vi "Laser Device Control.vi"(7 "Calling VI Ref":refnum<vi>) -> ()   [LabVIEW 2020]
uses:
  Laser Device Control Type Defs/Laser Device Control Control.ctl
  Hardware Configuration/Hardware Configuration Controls/Device Type.ctl
  <vilib>/Utility/miscctls.llb/LVPointTypeDef.ctl
  Device Library/Lasers/Laser Controls/Laser Actions.ctl
  Device Manager/Common Device Queue/Common Device Controls/Common Device Actions.ctl
  <vilib>/regexp/Match Regular Expression.xnode
panel:
  in  "Laser 05":T1={"Wavelength (nm)"=0, "Connect Text"="", "Connection"=TRUE, "Laser Status"="", "Emission"=TRUE, "Power (mW)"=0.0, "Settings"=TRUE}
  in  "Laser 04":T1={"Wavelength (nm)"=0, "Connect Text"="", "Connection"=TRUE, "Laser Status"="", "Emission"=TRUE, "Power (mW)"=0.0, "Settings"=TRUE}
  in  "Laser 03":T1={"Wavelength (nm)"=0, "Connect Text"="", "Connection"=TRUE, "Laser Status"="", "Emission"=TRUE, "Power (mW)"=0.0, "Settings"=TRUE}
  in  "Laser 02":T1={"Wavelength (nm)"=0, "Connect Text"="", "Connection"=TRUE, "Laser Status"="", "Emission"=TRUE, "Power (mW)"=0.0, "Settings"=TRUE}
  in  "Laser 01":T1={"Wavelength (nm)"=0, "Connect Text"="", "Connection"=TRUE, "Laser Status"="", "Emission"=TRUE, "Power (mW)"=0.0, "Settings"=TRUE}
  in  "Quit":bool
  # "Status:"
  # "Status:"
  # "Status:"
  # "Status:"
  # "Status:"
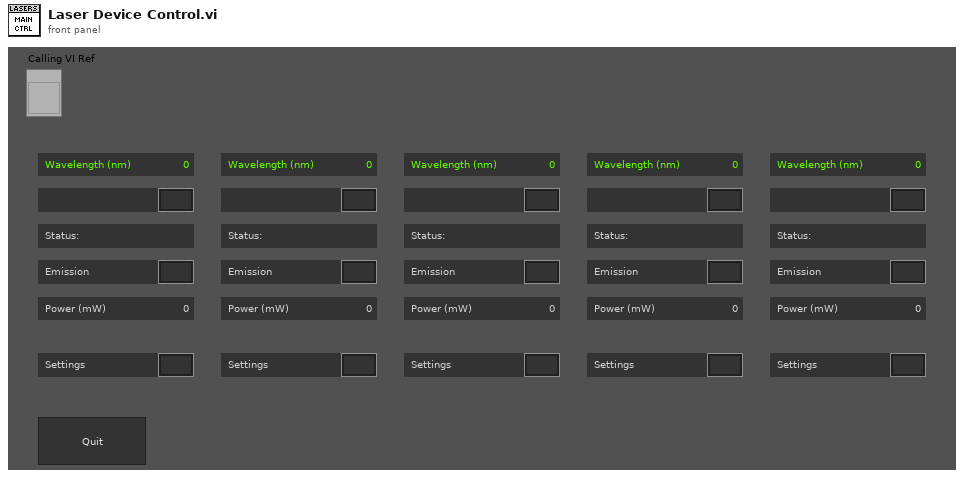
[diagram p1: front panel]
types:
  T1 = typedef "Laser Device Control Control.ctl" = cluster{"Wavelength (nm)":u16, "Connect Text":string, "Connection":bool, "Laser Status":string, "Emission":bool, "Power (mW)":dbl, "Settings":bool}
  T2 = enum16{"Always On", "Always Off", "Off While Running"}
  T3 = typedef "LVPointTypeDef.ctl" = cluster{"Horizontal":i16, "Vertical":i16}
  T4 = typedef "Device Type.ctl" = enum16{"AOTF", "Camera", "Deformable Mirror", "Laser", "Microscope Base", "Shutter", "Stage", "Waveform", "FPGA", "Email", "Filter Wheel", "Spinning Disk"}
  T5 = typedef "LVRectTypeDef.ctl" = cluster{"Left":i16, "Top":i16, "Right":i16, "Bottom":i16}
  T6 = typedef "LVBoundsTypeDef.ctl" = cluster{"Width":u32, "Height":u32}
  T7 = typedef "Laser Actions.ctl" = enum16{"Error Check", "Set On/Off", "Set Power", "Set Parameter", "Get Power", "Get Status", "Get Parameter", "Quit"}
  T8 = typedef "Common Device Actions.ctl" = enum16{"Specific Action", "Open Front Panel", "Close Front Panel", "Quit", "Quit All"}
  T9 = typedef "Laser Control Control.ctl" = cluster{"Wavelength (nm)":u16, "Connect Text":string, "Connection":bool, "Laser Status":string, "Emission":bool, "Power (mW)":dbl, "Settings":bool}
  T10 = typedef "Device Function.ctl" = enum16{"Primary", "Secondary", "Overview", "Wide Field Drift Correction", "642 nm Excitation", "560 nm Excitation", "940 nm Excitation", "546 nm Excitation", "488 nm Excitation", "405 nm Excitation", "Objective Drift Correction", "4Pi Objective Lock", "Objective XY", "Objective Z", "Sample XY", "Sample Coarse Z", "Sample Z", "4Pi Lower", "4Pi Upper", "Mojo", "Adj Cavity", "Line Scanning", "Alert"}
  T11 = typedef "Laser Status.ctl" = enum16{"Warmup", "Ready", "Emission", "Tuning", "Error"}
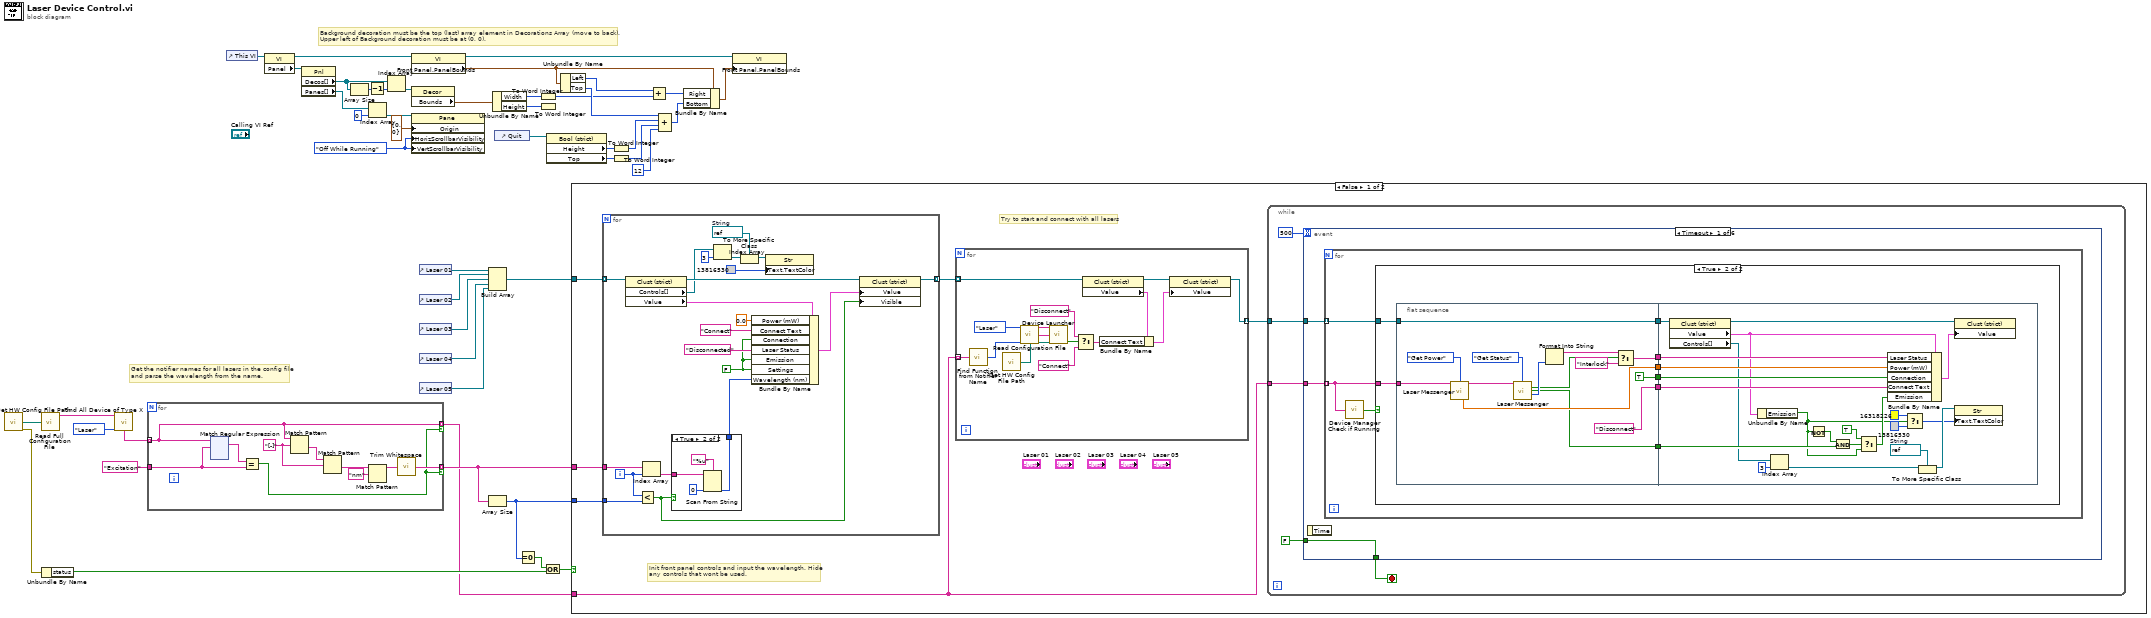
[diagram p0: block diagram]
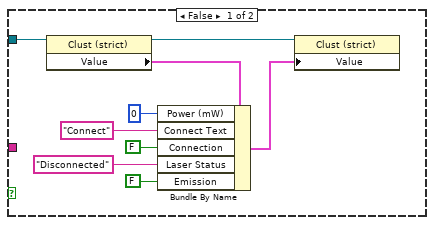
[diagram p2: hidden frame]
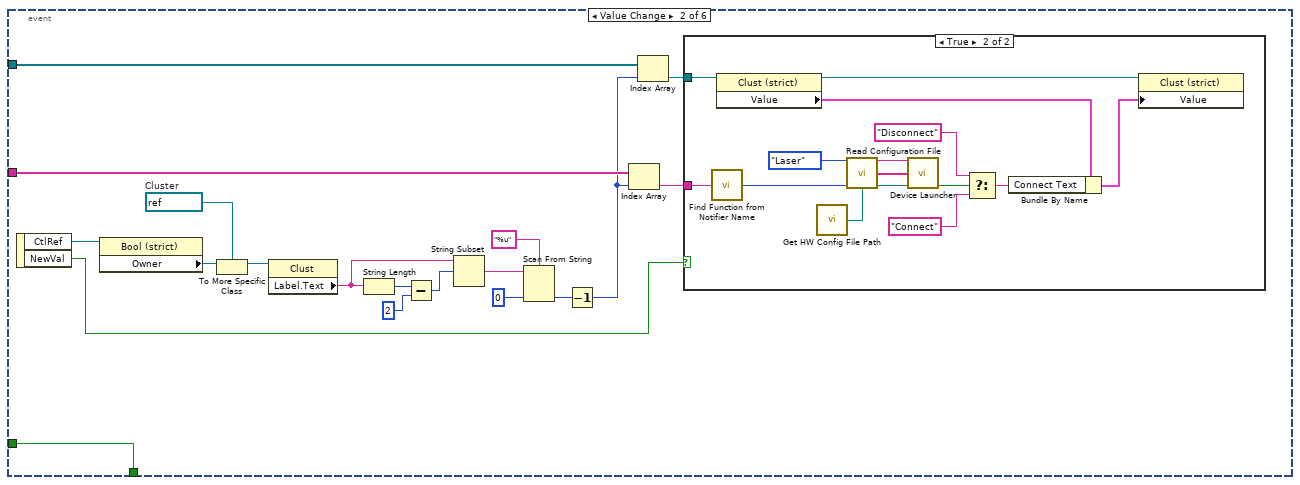
[diagram p3: hidden frame]
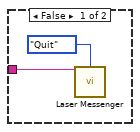
[diagram p4: hidden frame]
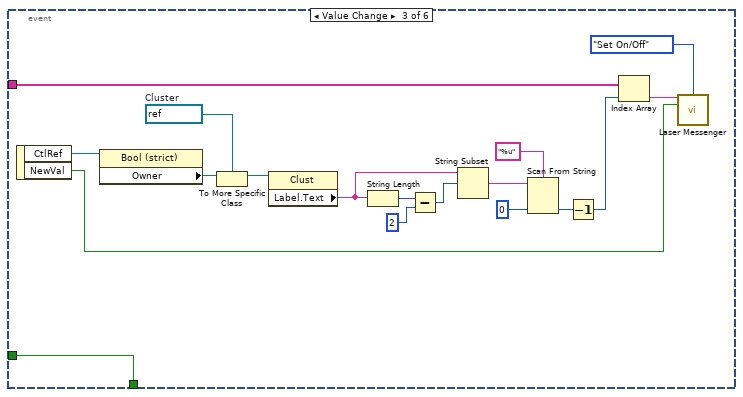
[diagram p5: hidden frame]
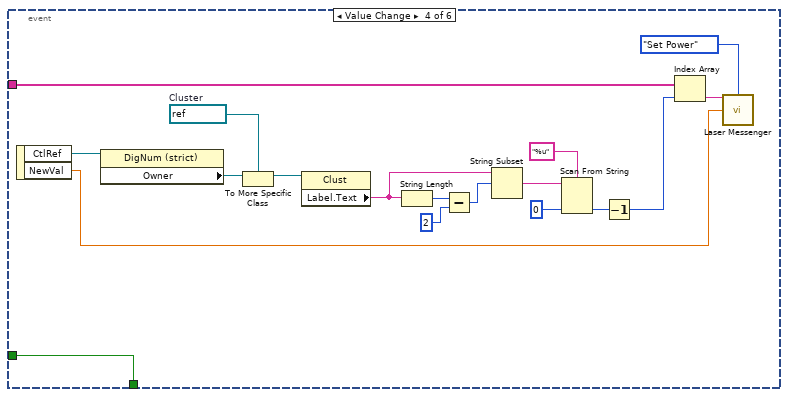
[diagram p6: hidden frame]
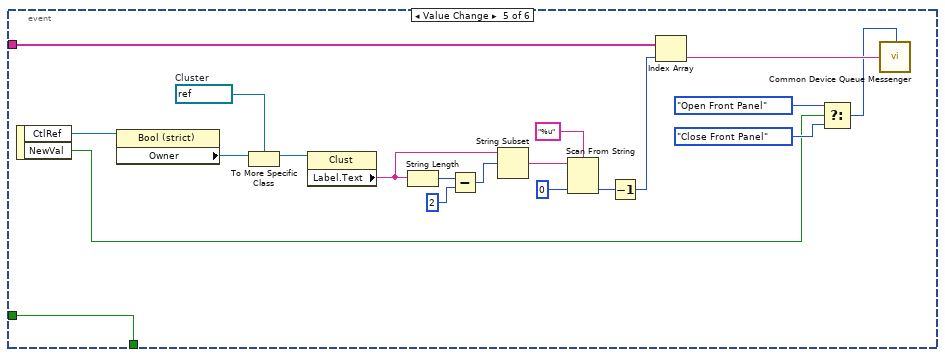
[diagram p7: hidden frame]
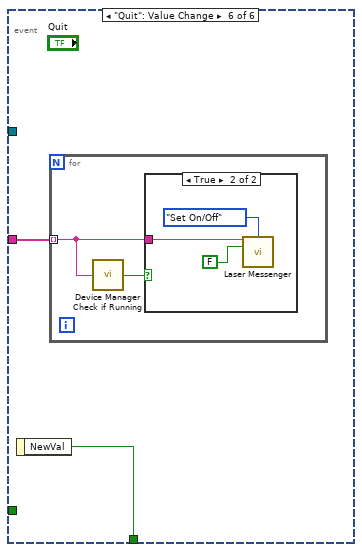
[diagram p8: hidden frame]
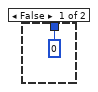
[diagram p10: hidden frame]
diagram:
  w27 = T2."Off While Running" ("Vertical Scrollbar Visibility")
  # "Get the notifier names for all lasers in the config file\nand parse the wavelength from the name."
  # "Background decoration must be the top (last) array element in Decorations Array (move to back).\nUpper left of Background decoration must be at (0, 0)."
  n1 = call "Get HW Config File Path.vi"() -> ("File Path"=w47:path, "Error"=w5:errorcluster)  [unwired: 14 in]
  n2 = call "Read Full Configuration File.vi"("Config File Path"=w47) -> ("Unique Notifier Names"=w46:string[])  [unwired: 11 in, 3 out]
  n3 = Unbundle By Name(w5) -> ("status"=w4:bool)
  n4 = call "Find All Device of Type X.vi"("Unique Notifier Names"=w46, "Device Type"=Device_Type."Laser") -> ("All Devices"=w10:string[])  [unwired: 12 in, 1 out]
  n5 = for {
    tunnel: w10 -> [w55] mode=indexing
    tunnel: [w55] -> w1 mode=indexing if=w48
    tunnel: "Excitation" -> [w56]
    tunnel: [w49] -> w3 mode=indexing if=w48
    w53 = "[-]" ("regular expression")
    n6 = xnode "Match Regular Expression"("input string"=w55, "regular expression"=w56) -> ("whole match"=w57:string)  [unwired: 4 in, 4 out]
    n7 = Equal?(x=w57, y=w56) -> (x = y?=w48:bool)
    n8 = Match Pattern(string=w55, regular expression=w53) -> (after substring=w54:string)  [unwired: 1 in, 3 out]
    n9 = Match Pattern(string=w54, regular expression=w53) -> (after substring=w52:string)  [unwired: 1 in, 3 out]
    n10 = Match Pattern(string=w52, regular expression="nm") -> (before substring=w50:string)  [unwired: 1 in, 3 out]
    n11 = call <vilib>:"Trim Whitespace.vi"("string"=w50) -> ("trimmed string"=w49:string)  [unwired: 1 in]
  }
  n12 = control-ref of="This VI"() -> (w19:refnum<vi>)
  n13 = property class="VI"(reference=w19) -> (reference out=w28:refnum<vi>, "Panel"=w20:refnum<vi>)  [unwired: 1 in, 1 out]
  n14 = property class="Pnl"(reference=w20) -> ("Decos[]"=w18:refnum<vi>[], "Panes[]"=w24:refnum<vi>[])  [unwired: 1 in, 2 out]
  n15 = Array Size(array=w18) -> (size(s)=w16:i32)
  n16 = Decrement(x=w16) -> (x-1=w17:i32)
  n17 = Index Array(array=w24, index=0) -> (element=w23:refnum<vi>)
  n18 = Index Array(array=w18, index=w17) -> (element=w26:refnum<vi>)
  n19 = property class="VI"(reference=w28) -> (reference out=w30:refnum<vi>, "Front Panel.PanelBounds"=w31:T5)  [unwired: 1 in, 1 out]
  n20 = property class="Decor"(reference=w26) -> ("Bounds"=w29:T6)  [unwired: 1 in, 2 out]
  n21 = property class="Pane"(reference=w23, "Origin"=T3 {"Horizontal"=0, "Vertical"=0}, "HorizScrollbarVisibility"=w27, "VertScrollbarVisibility"=w27) -> ()  [unwired: 1 in, 2 out]
  n22 = control-ref of="Laser 01"() -> (w15:refnum<vi>)
  n23 = control-ref of="Laser 02"() -> (w11:refnum<vi>)
  n24 = control-ref of="Laser 03"() -> (w12:refnum<vi>)
  n25 = control-ref of="Laser 04"() -> (w13:refnum<vi>)
  n26 = control-ref of="Laser 05"() -> (w14:refnum<vi>)
  n27 = Array Size(array=w3) -> (size(s)=w7:i32)
  n28 = Build Array(w15, w11, w12, w13, w14) -> (w8:refnum<vi>[])
  n29 = Unbundle By Name(w29) -> ("Width"=w34:u32, "Height"=w37:u32)
  n30 = control-ref of="Quit"() -> (w21:refnum<vi>)
  n31 = Equal To 0?(x=w7) -> (x = 0?=w6:bool)
  n32 = To Word Integer(number=w34) -> (16bit integer=w36:i16)
  n33 = To Word Integer(number=w37) -> ()  [unwired: 1 out]
  n34 = Or(x=w6, y=w4) -> (x .or. y?=w2:bool)
  n35 = property class="Bool (strict)"(reference=w21) -> ("Height"=w39:u32, "Top"=w40:i32)  [unwired: 1 in, 2 out]
  n36 = Unbundle By Name(w31) -> ("Left"=w33:i16, "Top"=w44:i16)
  n37 = case shown="False" w2 {
    tunnel: w8 -> [w177 _]
    tunnel: w7 -> [w176 _]
    tunnel: w3 -> [w175 _]
    tunnel: w1 -> [w172 _]
    frame False {
      # "Try to start and connect with all lasers"
      # "Init front panel controls and input the wavelength. Hide\nany controls that wont be used."
      n38 = for {
        tunnel: w177 -> [w377] mode=indexing
        tunnel: w175 -> [w369]
        tunnel: [w370] -> w174 mode=indexing
        tunnel: w176 -> [w367]
        i -> [w368]
        w360 = refnum<vi> refnum  # String
        w363 = FALSE ("Settings")
        n39 = property class="Clust (strict)"(reference=w377) -> (reference out=w374:refnum<vi>, "Controls[]"=w359:refnum<vi>[], "Value"=w376:T9)  [unwired: 1 in, 1 out]
        n40 = Less?(x=w368, y=w367) -> (x < y?=w365:bool)
        n41 = Index Array(array=w369, index=w368) -> (element=w366:string)
        n42 = case shown="True" w365 {
          tunnel: [u16 0 ("default value 1") w380] -> w364
          tunnel: w366 -> [_ w379]
          frame False {
          }
          frame True {
            n43 = Scan From String(format string="%u", input string=w379, default 1=u16 0 ("default value 1")) -> (output 1=w380:u16)  [unwired: 2 in, 3 out]
          }
        }
        n44 = Index Array(array=w359, index=3) -> (element=w357:refnum<vi>)
        n45 = To More Specific Class(target class=w360, reference=w357) -> (specific class reference=w361:refnum<vi>)  [unwired: 1 in, 1 out]
        n46 = Bundle By Name(cluster=w376, "Power (mW)"=0.0, "Connect Text"="Connect", "Connection"=w363, "Laser Status"="Disconnected", "Emission"=w363, "Settings"=w363, "Wavelength (nm)"=w364) -> (w373:T9)
        n47 = property class="Str"(reference=w361, "Text.TextColor"=u32 13816530) -> ()  [unwired: 1 in, 2 out]
        n48 = property class="Clust (strict)"(reference=w374, "Value"=w373, "Visible"=w365) -> (reference out=w370:refnum<vi>)  [unwired: 1 in, 1 out]
      }
      n49 = for {
        tunnel: w174 -> [w180] mode=indexing
        tunnel: [w179] -> w173 mode=indexing
        tunnel: w172 -> [w178] mode=indexing
        n50 = call "Find Function from Notifier Name.vi"("Unique Notifier Name"=w178) -> ("Function"=w193:T10)  [unwired: 14 in]
        n51 = call "Get HW Config File Path.vi"() -> ("File Path"=w182:path)  [unwired: 14 in, 1 out]
        n52 = call "Read Configuration File.vi"("Device Type"=Device_Type."Laser", "Device Function"=w193, "Config File Path"=w182) -> ("Unique Notifier Name"=w183:string, "Device Ports/IDs/Channels"=w185:string[], "Device Engine Path"=w184:path)  [unwired: 9 in, 1 out]
        n53 = call "Device Launcher.vi"("Notifier Name"=w183, "Device Ports/IDs/Channels"=w185, "Device Engine Path"=w184) -> ("Running?"=w187:bool)  [unwired: 11 in, 1 out]
        n54 = Select(t="Disconnect", s=w187, f="Connect") -> (s? t:f=w190:string)
        n55 = property class="Clust (strict)"(reference=w180) -> (reference out=w191:refnum<vi>, "Value"=w186:T9)  [unwired: 1 in, 1 out]
        n56 = Bundle By Name(cluster=w186, "Connect Text"=w190) -> (w192:T9)
        n57 = property class="Clust (strict)"(reference=w191, "Value"=w192) -> (reference out=w179:refnum<vi>)  [unwired: 1 in, 1 out]
      }
      n58 = while {
        tunnel: w172 -> [w197]
        tunnel: w173 -> [w196]
        stop <- w195 stop-if-true
        n59 = event shown="[0] Timeout" {
          selector: _ -> [_ _ _ _ _ _]
          dyn-events: _ -> [_ _ _ _ _ _]
          timeout: 500 -> [_ _ _ _ _ _]
          tunnel: w197 -> [w201 w269 w303 w321 w334 w350]
          tunnel: w196 -> [w200 w267 _ _ _ _]
          tunnel: [w199 w276 w311 w329 w349 w351] -> w195
          tunnel: FALSE -> [w199 w276 w311 w329 w349 _]
          event Timeout {
            n60 = event-data() -> ()  [unwired: 1 in, 1 out]
            n61 = for {
              tunnel: w201 -> [w203] mode=indexing
              tunnel: w200 -> [w204] mode=indexing
              n62 = call "Device Manager Check if Running.vi"("Notifier Name"=w203) -> ("Running?"=w202:bool)  [unwired: 14 in]
              n63 = case shown="True" w202 {
                tunnel: w204 -> [w213 w215]
                tunnel: w203 -> [_ w221]
                frame False {
                  n64 = property class="Clust (strict)"(reference=w213) -> (reference out=w206:refnum<vi>, "Value"=w207:T9)  [unwired: 1 in, 1 out]
                  n65 = Bundle By Name(cluster=w207, "Power (mW)"=u16 0, "Connect Text"="Connect", "Connection"=FALSE, "Laser Status"="Disconnected", "Emission"=FALSE) -> (w205:T9)
                  n66 = property class="Clust (strict)"(reference=w206, "Value"=w205) -> ()  [unwired: 1 in, 2 out]
                }
                frame True {
                  n67 = flat-sequence {
                    tunnel: w221 -> [w227]
                    tunnel: [w230] -> w220
                    tunnel: [w226] -> w219
                    tunnel: ["Disconnect" ("Connect Text")] -> w218
                    tunnel: [TRUE ("Connection")] -> w217
                    tunnel: [w223] -> w216
                    tunnel: w215 -> [w223]
                    tunnel: [w222] -> w214
                    tunnel: w220 -> [w255]
                    tunnel: w219 -> [w254]
                    tunnel: w218 -> [w252]
                    tunnel: w217 -> [w253]
                    tunnel: w216 -> [w251]
                    tunnel: w214 -> [w249]
                    frame #0 {
                      n68 = call "Laser Messenger.vi"("Notifier Name"=w227, "Action"=Laser_Actions."Get Power") -> ("Notifier Name Dup"=w229:string, "Power (mW)"=w226:dbl)  [unwired: 8 in, 4 out]
                      n69 = call "Laser Messenger.vi"("Notifier Name"=w229, "Action"=Laser_Actions."Get Status") -> ("Enabled (Interlock)?"=w233:bool, "Light Emission?"=w222:bool, "Laser Status"=w234:T11)  [unwired: 8 in, 3 out]
                      n70 = Format Into String(w234) -> (resulting string=w232:string)  [unwired: 3 in, 1 out]
                      n71 = Select(t=w232, s=w233, f="Interlock") -> (s? t:f=w230:string)
                    }
                    frame #1 {
                      w242 = refnum<vi> refnum  # String
                      n72 = property class="Clust (strict)"(reference=w251) -> (reference out=w257:refnum<vi>, "Value"=w250:T9, "Controls[]"=w244:refnum<vi>[])  [unwired: 1 in, 1 out]
                      n73 = Unbundle By Name(w250) -> ("Emission"=w239:bool)
                      n74 = Index Array(array=w244, index=3) -> (element=w236:refnum<vi>)
                      n75 = Not(x=w239) -> (.not. x?=w248:bool)
                      n76 = And(x=w248, y=w249) -> (x .and. y?=w247:bool)
                      n77 = Select(t=TRUE, s=w247, f=w239) -> (s? t:f=w245:bool)
                      n78 = Bundle By Name(cluster=w250, "Laser Status"=w255, "Power (mW)"=w254, "Connection"=w253, "Connect Text"=w252, "Emission"=w245) -> (w256:T9)
                      n79 = Select(t=u32 16318226 ("Color Box"), s=w239, f=u32 13816530) -> (s? t:f=w237:u32)
                      n80 = To More Specific Class(target class=w242, reference=w236) -> (specific class reference=w241:refnum<vi>)  [unwired: 1 in, 1 out]
                      n81 = property class="Str"(reference=w241, "Text.TextColor"=w237) -> ()  [unwired: 1 in, 2 out]
                      n82 = property class="Clust (strict)"(reference=w257, "Value"=w256) -> ()  [unwired: 1 in, 2 out]
                    }
                  }
                }
              }
            }
          }
          event Value Change {
            w263 = refnum<vi> refnum  # Cluster
            n83 = event-data() -> ("CtlRef"=w261:refnum<vi>, "NewVal"=w258:bool)  [unwired: 1 in]
            n84 = property class="Bool (strict)"(reference=w261) -> ("Owner"=w262:refnum<vi>)  [unwired: 1 in, 2 out]
            n85 = To More Specific Class(target class=w263, reference=w262) -> (specific class reference=w264:refnum<vi>)  [unwired: 1 in, 1 out]
            n86 = property class="Clust"(reference=w264) -> ("Label.Text"=w260:string)  [unwired: 1 in, 2 out]
            n87 = String Length(string=w260) -> (length=w275:i32)
            n88 = Subtract(x=w275, y=2) -> (x-y=w273:i32)
            n89 = String Subset(string=w260, offset (0)=w273) -> (substring=w270:string)  [unwired: 1 in]
            n90 = Scan From String(format string="%u", input string=w270, default 1=0) -> (output 1=w266:i32)  [unwired: 2 in, 3 out]
            n91 = Decrement(x=w266) -> (x-1=w259:i32)
            n92 = Index Array(array=w269, index=w259) -> (element=w268:string)
            n93 = Index Array(array=w267, index=w259) -> (element=w265:refnum<vi>)
            n94 = case shown="True" w258 {
              tunnel: w268 -> [w277 w288]
              tunnel: w265 -> [_ w286]
              frame False {
                n95 = call "Laser Messenger.vi"("Notifier Name"=w277, "Action"=Laser_Actions."Quit") -> ()  [unwired: 8 in, 6 out]
              }
              frame True {
                n96 = call "Find Function from Notifier Name.vi"("Unique Notifier Name"=w288) -> ("Function"=w287:T10)  [unwired: 14 in]
                n97 = property class="Clust (strict)"(reference=w286) -> (reference out=w280:refnum<vi>, "Value"=w285:T9)  [unwired: 1 in, 1 out]
                n98 = call "Get HW Config File Path.vi"() -> ("File Path"=w292:path)  [unwired: 14 in, 1 out]
                n99 = call "Read Configuration File.vi"("Device Type"=Device_Type."Laser", "Device Function"=w287, "Config File Path"=w292) -> ("Unique Notifier Name"=w291:string, "Device Ports/IDs/Channels"=w289:string[], "Device Engine Path"=w290:path)  [unwired: 9 in, 1 out]
                n100 = call "Device Launcher.vi"("Notifier Name"=w291, "Device Ports/IDs/Channels"=w289, "Device Engine Path"=w290) -> ("Running?"=w284:bool)  [unwired: 11 in, 1 out]
                n101 = Select(t="Disconnect", s=w284, f="Connect") -> (s? t:f=w281:string)
                n102 = Bundle By Name(cluster=w285, "Connect Text"=w281) -> (w279:T9)
                n103 = property class="Clust (strict)"(reference=w280, "Value"=w279) -> ()  [unwired: 1 in, 2 out]
              }
            }
          }
          event Value Change {
            w299 = refnum<vi> refnum  # Cluster
            n104 = event-data() -> ("CtlRef"=w297:refnum<vi>, "NewVal"=w295:bool)  [unwired: 1 in]
            n105 = property class="Bool (strict)"(reference=w297) -> ("Owner"=w298:refnum<vi>)  [unwired: 1 in, 2 out]
            n106 = To More Specific Class(target class=w299, reference=w298) -> (specific class reference=w300:refnum<vi>)  [unwired: 1 in, 1 out]
            n107 = property class="Clust"(reference=w300) -> ("Label.Text"=w296:string)  [unwired: 1 in, 2 out]
            n108 = String Length(string=w296) -> (length=w310:i32)
            n109 = Subtract(x=w310, y=2) -> (x-y=w308:i32)
            n110 = String Subset(string=w296, offset (0)=w308) -> (substring=w305:string)  [unwired: 1 in]
            n111 = Scan From String(format string="%u", input string=w305, default 1=0) -> (output 1=w304:i32)  [unwired: 2 in, 3 out]
            n112 = Decrement(x=w304) -> (x-1=w294:i32)
            n113 = Index Array(array=w303, index=w294) -> (element=w302:string)
            n114 = call "Laser Messenger.vi"("Notifier Name"=w302, "Action"=Laser_Actions."Set On/Off", "Emission On/Off"=w295) -> ()  [unwired: 7 in, 6 out]
          }
          event Value Change {
            w316 = refnum<vi> refnum  # Cluster
            n115 = event-data() -> ("CtlRef"=w314:refnum<vi>, "NewVal"=w318:dbl)  [unwired: 1 in]
            n116 = property class="DigNum (strict)"(reference=w314) -> ("Owner"=w315:refnum<vi>)  [unwired: 1 in, 2 out]
            n117 = To More Specific Class(target class=w316, reference=w315) -> (specific class reference=w317:refnum<vi>)  [unwired: 1 in, 1 out]
            n118 = property class="Clust"(reference=w317) -> ("Label.Text"=w313:string)  [unwired: 1 in, 2 out]
            n119 = String Length(string=w313) -> (length=w328:i32)
            n120 = Subtract(x=w328, y=2) -> (x-y=w326:i32)
            n121 = String Subset(string=w313, offset (0)=w326) -> (substring=w323:string)  [unwired: 1 in]
            n122 = Scan From String(format string="%u", input string=w323, default 1=0) -> (output 1=w322:i32)  [unwired: 2 in, 3 out]
            n123 = Decrement(x=w322) -> (x-1=w312:i32)
            n124 = Index Array(array=w321, index=w312) -> (element=w320:string)
            n125 = call "Laser Messenger.vi"("Notifier Name"=w320, "Action"=Laser_Actions."Set Power", "Power (mW)"=w318) -> ()  [unwired: 7 in, 6 out]
          }
          event Value Change {
            w338 = refnum<vi> refnum  # Cluster
            n126 = event-data() -> ("CtlRef"=w335:refnum<vi>, "NewVal"=w331:bool)  [unwired: 1 in]
            n127 = property class="Bool (strict)"(reference=w335) -> ("Owner"=w337:refnum<vi>)  [unwired: 1 in, 2 out]
            n128 = To More Specific Class(target class=w338, reference=w337) -> (specific class reference=w339:refnum<vi>)  [unwired: 1 in, 1 out]
            n129 = property class="Clust"(reference=w339) -> ("Label.Text"=w336:string)  [unwired: 1 in, 2 out]
            n130 = String Length(string=w336) -> (length=w346:i32)
            n131 = Subtract(x=w346, y=2) -> (x-y=w344:i32)
            n132 = String Subset(string=w336, offset (0)=w344) -> (substring=w341:string)  [unwired: 1 in]
            n133 = Scan From String(format string="%u", input string=w341, default 1=0) -> (output 1=w340:i32)  [unwired: 2 in, 3 out]
            n134 = Decrement(x=w340) -> (x-1=w333:i32)
            n135 = Index Array(array=w334, index=w333) -> (element=w332:string)
            n136 = Select(t=Common_Device_Actions."Open Front Panel" ("Common Actions"), s=w331, f=Common_Device_Actions."Close Front Panel" ("Common Actions")) -> (s? t:f=w330:T8)
            n137 = call "Common Device Queue Messenger.vi"("Common Action"=w330, "Notifier Name"=w332) -> ()  [unwired: 13 in, 1 out]
          }
          event "Quit": Value Change {
            n138 = event-data() -> ("NewVal"=w351:bool)  [unwired: 1 in]
            n139 = for {
              tunnel: w350 -> [w353] mode=indexing
              n140 = call "Device Manager Check if Running.vi"("Notifier Name"=w353) -> ("Running?"=w352:bool)  [unwired: 14 in]
              n141 = case shown="True" w352 {
                tunnel: w353 -> [_ w354]
                frame False {
                }
                frame True {
                  n142 = call "Laser Messenger.vi"("Notifier Name"=w354, "Action"=Laser_Actions."Set On/Off", "Emission On/Off"=FALSE) -> ()  [unwired: 7 in, 6 out]
                }
              }
            }
          }
        }
      }
    }
    frame True {
    }
  }
  n143 = To Word Integer(number=w39) -> (16bit integer=w42:i16)
  n144 = To Word Integer(number=w40) -> (16bit integer=w43:i16)
  n145 = Add(x=w33, y=w36) -> (x+y=w35:i16)
  n146 = Compound Arithmetic op=ADD(w44, w42, w43, i16 12 ("y")) -> (w38:i16)
  n147 = Bundle By Name(cluster=w31, "Right"=w35, "Bottom"=w38) -> (w32:T5)
  n148 = property class="VI"(reference=w30, "Front Panel.PanelBounds"=w32) -> ()  [unwired: 1 in, 2 out]
